vi "ACL_Read_Plot.vi"(8 "error in (no error)":errorcluster, 10 "PmodACL address":u8, 11 "I2C Ref Out":T1) -> (0 "error out":errorcluster, 1 "Numeric 3":i16, 2 "Array":bool[](array[boolean]), 3 "Numeric":i16, 4 "Cluster":cluster{i16, i16, i16}, 5 "Numeric 2":i16)   [LabVIEW 2021]
uses:
  <vilib>/myRIO/Instrument Drivers/Onboard IO/I2C/typedefs/I2C Reference.ctl
  <vilib>/myRIO/Common/Instrument Driver Framework/Utilities/typedefs/myRIO Generic Hardware Reference.ctl
  <vilib>/myRIO/Common/Instrument Driver Framework/Utilities/typedefs/Hardware Version Enum.ctl
  <vilib>/myRIO/Common/Instrument Driver Framework/Utilities/typedefs/myRIO v1.0 Reference.ctl
  <vilib>/myRIO/Common/Instrument Driver Framework/Utilities/typedefs/Generic FPGA Reference.ctl
  <vilib>/myRIO/Common/Instrument Driver Framework/myRIO v1.0/I2C/typedefs/I2C Channels Enum.ctl
  <vilib>/myRIO/Instrument Drivers/Onboard IO/I2C/typedefs/I2C Configuration.ctl
  <vilib>/myRIO/Instrument Drivers/Onboard IO/I2C/typedefs/I2C Transfer Rate.ctl
  <vilib>/Utility/error.llb/Error Cluster From Error Code.vi
  <vilib>/myRIO/Common/Instrument Driver Framework/myRIO v1.0/I2C/vis/myRIO v1.0 Write I2C.vi
  <vilib>/myRIO/Common/Instrument Driver Framework/myRIO v1.0/I2C/vis/myRIO v1.0 Read I2C.vi
  <vilib>/myRIO/Instrument Drivers/Onboard IO/I2C/I2C.lvlib
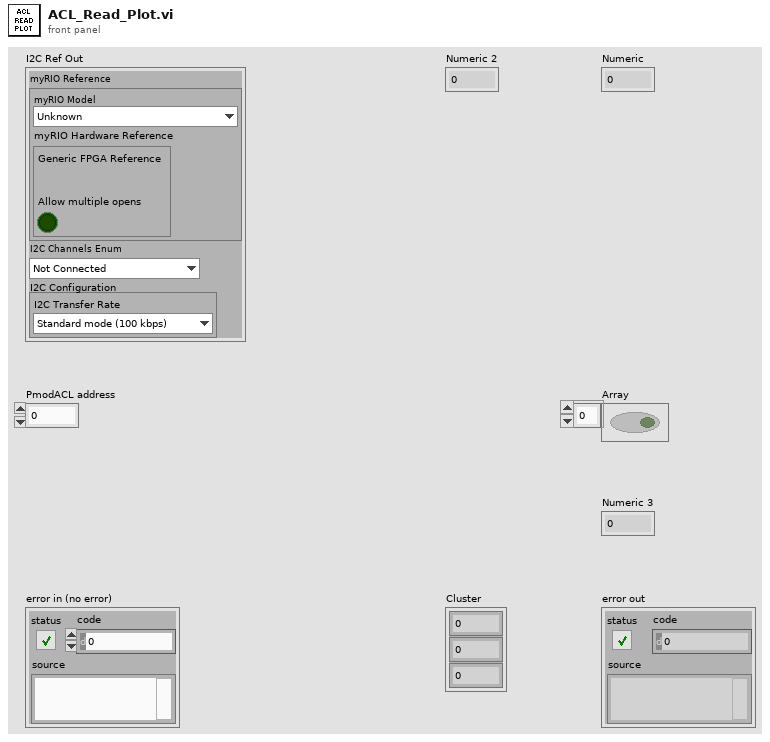
[diagram p1: front panel]
types:
  T1 = typedef "I2C.lvlib/I2C Reference.ctl" = cluster{"myRIO Reference":T2, "I2C Channels Enum":T6, "I2C Configuration":T7}
  T2 = typedef "myRIO Generic Hardware Reference.ctl" = cluster{"myRIO Model":T3, "myRIO Hardware Reference":T4}
  T3 = typedef "Hardware Version Enum.ctl" = enum16{"Unknown", "myRIO-1900", "myRIO-1950", "roboRIO", "NI ELVIS RIO CM", "ELVIS III"}
  T4 = typedef "myRIO v1.0 Reference.ctl" = cluster{"Generic FPGA Reference":T5, "Allow multiple opens":bool}
  T5 = typedef "Generic FPGA Reference.ctl" = refnum<k20>
  T6 = typedef "I2C Channels Enum.ctl" = enum16{"Not Connected", "A/I2C", "B/I2C", "I2C/I2C"}
  T7 = typedef "I2C.lvlib/I2C Configuration.ctl" = cluster{"I2C Transfer Rate":T8}
  T8 = typedef "I2C.lvlib/I2C Transfer Rate.ctl" = enum16{"Standard mode (100 kbps)", "Fast mode (400 kbps)"}
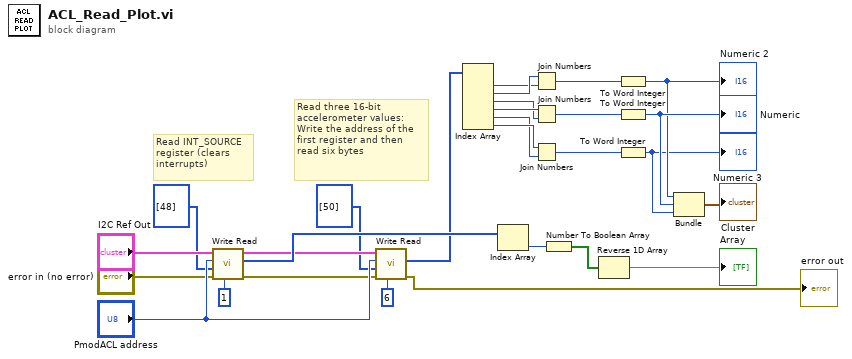
[diagram p0: block diagram]
diagram:
  # "Read INT_SOURCE\nregister (clears\ninterrupts)"
  # "Read three 16-bit accelerometer values:\nWrite the address of the first register and then read six bytes"
  n1 = call <vilib>:"Write Read.vi"("Byte Count"=u32 1, "error in (no error)"="error in (no error)", "Bytes to Write"=u8[] [48], "Slave Address (7-bit)"="PmodACL address", "I2C Ref In"="I2C Ref Out") -> ("error out"=w21:errorcluster, "Bytes Read"=w28:u8[], "I2C Ref Out"=w20:T1)  [unwired: 3 in]
  n2 = call <vilib>:"Write Read.vi"("Byte Count"=u32 6, "error in (no error)"=w21, "Bytes to Write"=u8[] [50], "Slave Address (7-bit)"="PmodACL address", "I2C Ref In"=w20) -> ("error out"=→"error out":errorcluster, "Bytes Read"=w27:u8[])  [unwired: 3 in, 1 out]
  n3 = Index Array "Index Array"(array=w27) -> (element #1=w12:u8, element #2=w13:u8, element #3=w14:u8, element #4=w15:u8, element #5=w16:u8, element #6=w17:u8)  [unwired: 6 in]
  n4 = Index Array "Index Array"(array=w28) -> (element=w23:u8)  [unwired: 1 in]
  n5 = Join Numbers(hi=w13, lo=w12) -> ((hi.lo)=w1:u16)
  n6 = Join Numbers(hi=w15, lo=w14) -> ((hi.lo)=w2:u16)
  n7 = Join Numbers(hi=w17, lo=w16) -> ((hi.lo)=w3:u16)
  n8 = Number To Boolean Array(number=w23) -> (Boolean array=w24:bool[])
  n9 = Reverse 1D Array(array=w24) -> (reversed array=→"Array":bool[])
  n10 = To Word Integer(number=w1) -> (16bit integer=w6:i16)
  "Numeric 2" <- w6
  n11 = To Word Integer(number=w2) -> (16bit integer=w7:i16)
  "Numeric" <- w7
  n12 = To Word Integer(number=w3) -> (16bit integer=w4:i16)
  "Numeric 3" <- w4
  n13 = Bundle "Bundle"(w6, w7, w4) -> (→"Cluster":cluster{i16, i16, i16})  [unwired: 1 in]
